vi "accessfuncs.vi"() -> ()   [LabVIEW 2013]
panel:
  out "lvDataCluster.h":string="int writeDoubleElement(lvdatacluster*, int32, double*);\nint readDoubleElement(lvdatacluster*, int32, double*);\nint writeDoubleArrayElement(lvdatacluster*, int32, DoubleArrayHandle*);\nint readDoubleArrayElement(lvdatacluster*, int32, DoubleArrayHandle*);\nint writeSingleElement(lvdatacluster*, int32, float*);\nint readSingleElement(lvdatacluster*, int32, float*);\nint writeSingleArrayElement(lvdatacluster*, int32, SingleArrayHandle*);\nint readSingleArrayElement(lvdatacluster*, int32, SingleArrayHandle*);\nint writeI64Element(lvdatacluster*, int32, int64*);\nint readI64Element(lvdatacluster*, int32, int64*);\nint writeI64ArrayElement(lvdatacluster*, int32, I64ArrayHandle*);\nint readI64ArrayElement(lvdatacluster*, int32, I64ArrayHandle*);\nint writeI32Element(lvdatacluster*, int32, int32*);\nint readI32Element(lvdatacluster*, int32, int32*);\nint writeI32ArrayElement(lvdatacluster*, int32, I32ArrayHandle*);\nint readI32ArrayElement(lvdatacluster*, int32, I32ArrayHandle*);\nint writeI16Element(lvdatacluster*, int32, int16*);\nint readI16Element(lvdatacluster*, int32, int16*);\nint writeI16ArrayElement(lvdatacluster*, int32, I16ArrayHandle*);\nint readI16ArrayElement(lvdatacluster*, int32, I16ArrayHandle*);\nint writeI8Element(lvdatacluster*, int32, int8*);\nint readI8Element(lvdatacluster*, int32, int8*);\nint writeI8ArrayElement(lvdatacluster*, int32, I8ArrayHandle*);\nint readI8ArrayElement(lvdatacluster*, int32, I8ArrayHandle*);\nint writeU64Element(lvdatacluster*, int32, uInt64*);\nint readU64Element(lvdatacluster*, int32, uInt64*);\nint writeU64ArrayElement(lvdatacluster*, int32, U64ArrayHandle*);\nint readU64ArrayElement(lvdatacluster*, int32, U64ArrayHandle*);\nint writeU32Element(lvdatacluster*, int32, uInt32*);\nint readU32Element(lvdatacluster*, int32, uInt32*);\nint writeU32ArrayElement(lvdatacluster*, int32, U32ArrayHandle*);\nint readU32ArrayElement(lvdatacluster*, int32, U32ArrayHandle*);\nint writeU16Element(lvdatacluster*, int32, uInt16*);\nint readU16Element(lvdatacluster*, int32, uInt16*);\nint writeU16ArrayElement(lvdatacluster*, int32, U16ArrayHandle*);\nint readU16ArrayElement(lvdatacluster*, int32, U16ArrayHandle*);\nint writeU8Element(lvdatacluster*, int32, uInt8*);\nint readU8Element(lvdatacluster*, int32, uInt8*);\nint writeU8ArrayElement(lvdatacluster*, int32, U8ArrayHandle*);\nint readU8ArrayElement(lvdatacluster*, int32, U8ArrayHandle*);\nint writeBooleanElement(lvdatacluster*, int32, LVBoolean*);\nint readBooleanElement(lvdatacluster*, int32, LVBoolean*);\nint writeBooleanArrayElement(lvdatacluster*, int32, BooleanArrayHandle*);\nint readBooleanArrayElement(lvdatacluster*, int32, BooleanArrayHandle*);\nint writeStringElement(lvdatacluster*, int32, LStrHandle*);\nint readStringElement(lvdatacluster*, int32, LStrHandle*);\nint writeStringArrayElement(lvdatacluster*, int32, StringArrayHandle*);\nint readStringArrayElement(lvdatacluster*, int32, StringArrayHandle*);\n"
  in  "names":string[](array[string])=["Double", "Single", "I64", "I32", "I16", "I8", "U64", "U32", "U16", "U8", "Boolean", "String"]
  in  "types":string[](array[string])=["double", "float", "int64", "int32", "int16", "int8", "uInt64", "uInt32", "uInt16", "uInt8", "LVBoolean", "LStrHandle"]
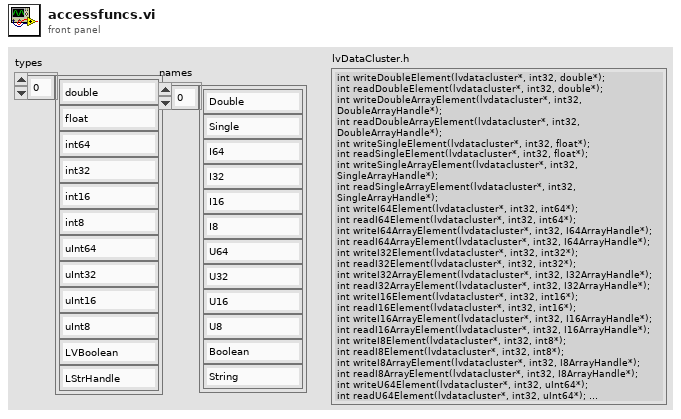
[diagram p1: front panel]
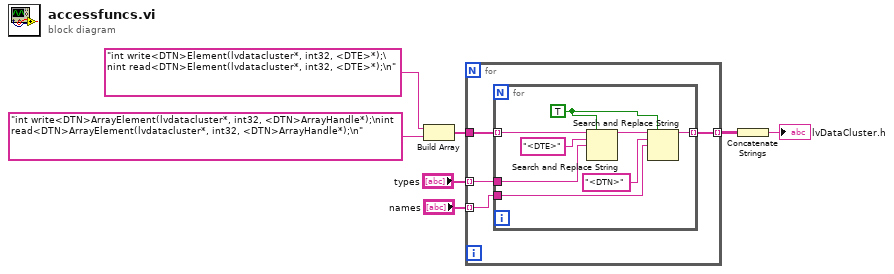
[diagram p0: block diagram]
diagram:
  n1 = Build Array("int write<DTN>Element(lvdatacluster*, int32, <DTE>*);\nint read<DTN>Element(lvdatacluster*, int32, <DTE>*);\n", "int write<DTN>ArrayElement(lvdatacluster*, int32, <DTN>ArrayHandle*);\nint read<DTN>ArrayElement(lvdatacluster*, int32, <DTN>ArrayHandle*);\n") -> (w1:string[])
  n2 = for {
    tunnel: "types" -> [w11] mode=indexing
    tunnel: "names" -> [w10] mode=indexing
    tunnel: w1 -> [w9]
    tunnel: [w8] -> w5 mode=indexing
    n3 = for {
      tunnel: w11 -> [w13]
      tunnel: w10 -> [w15]
      tunnel: w9 -> [w19] mode=indexing
      tunnel: [w17] -> w8 mode=indexing
      w12 = TRUE ("replace all? (F)")
      n4 = Search and Replace String(replace all?=w12, input string=w19, search string="<DTE>", replace string=w13) -> (result string=w18:string)  [unwired: 4 in, 3 out]
      n5 = Search and Replace String(replace all?=w12, input string=w18, search string="<DTN>", replace string=w15) -> (result string=w17:string)  [unwired: 4 in, 3 out]
    }
  }
  n6 = Concatenate Strings(w5) -> (→"lvDataCluster.h":string)
